vi "Module Cleanup.vi"(8 "error in (no error)":errorcluster, 11 "Role Manager in":refnum<class "Role Manager.lvclass">) -> (0 "error out":errorcluster, 3 "Role Manager out":refnum<class "Role Manager.lvclass">)   [LabVIEW 2020, in "Volatus.lvlib" / "Role Manager.lvclass"]
uses:
  Role Manager.lvclass
  Role Manager.lvclass/Role Manager.ctl
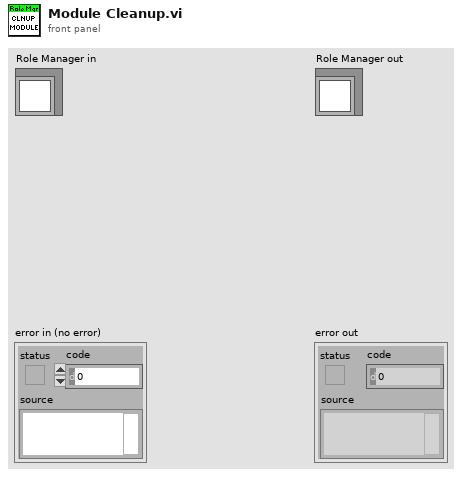
[diagram p1: front panel]
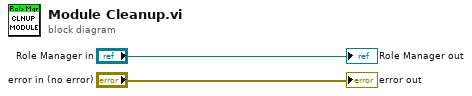
[diagram p0: block diagram]
diagram:
  "error out" <- "error in (no error)"
  "Role Manager out" <- "Role Manager in"
